vi "Test Report Contains Error Count.vi"(8 "error in (no error)":errorcluster, 11 "Text Report Test in":refnum<class "Text Report Test.lvclass">) -> (0 "error out":errorcluster, 3 "Text Report Test out":refnum<class "Text Report Test.lvclass">)   [LabVIEW 2020, in "Text Report Test.lvclass"]
uses:
  Text Report Test.lvclass
  Test Doubles/Test Case Test Double/Methods.ctl
  Text Report Test.lvclass/Text Report Test.ctl
  source/Plugins/Text Report/Text Report.lvclass
  Test Doubles/Test Case Test Double/Test Case Test Double.lvclass
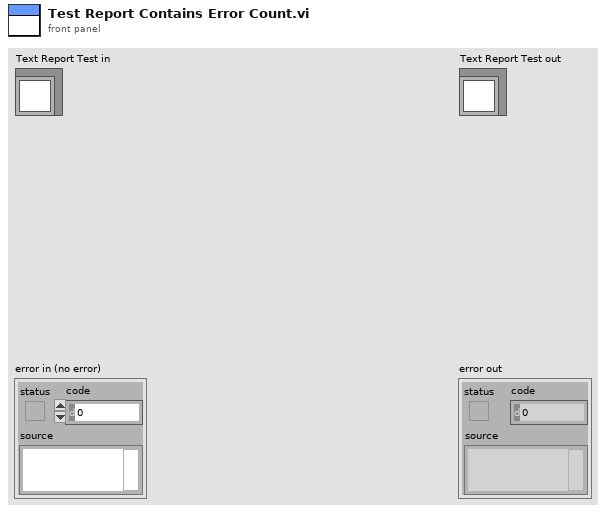
[diagram p1: front panel]
types:
  T1 = typedef "Test Case Test Double.lvclass/Methods.ctl" = enum16{"Test Failing Test.vi", "Test Passing Test.vi", "Test Error Test.vi", "Test Skip Test.vi", "Test Passing Pass If Test.vi", "Test Failing Pass If Test.vi", "Test Failing Fail If Test.vi", "Test Passing Fail If Test.vi", "Test Passing Pass If Error Test.vi", "Test Failing Pass If Error Test.vi", "Test Passing Fail If Error Test.vi", "Test Failing Fail If Error Test.vi", "Test Passing Pass If Equal Test.vi", "Test Failing Pass If Equal Test.vi", "Test Failing Fail If Equal Test.vi", "Test Passing Fail If Equal Test.vi", "Freezing Test.vi", "Test Pass on Expected Error Code.vi", "Test Error on Unexpected Error Code.vi", "Test Fail on Expected Error Code.vi", "Test Error when Fail on Unexpected Error Code.vi", "Test Pass on Expected Element in Array.vi", "Test Fail on Expected Element Not in Array.vi", "Test Pass on Expected Element in Set.vi", "Test Fail on Expected Element Not in Set.vi", "Test Pass on Expected Element in Map.vi", "Test Fail on Expected Element Not in Map.vi", "Test Fail on Unexpected Element in Array.vi", "Test Pass on Unexpected Element Not in Array.vi", "Test Fail if Unexpected Element in Set.vi", "Test Pass if Unexpected Element Not in Set.vi", "Test Fail if Unexpected Element in Map.vi", "Test Pass if Unexpected Element Not in Map.vi", "Test Pass on Expected Element in Array of Clusters.vi", "Test Pass on Expected Element Not in Array of Clusters.vi", "Test Matching String Test.vi", "Test Not Matching String Test.vi", "Verify Passing.vi", "Without Prefix.vi", "Private VI.vi"}
  T2 = typedef "Result.lvlib/Result.ctl" = cluster{"Name":string, "Description":string, "Status":T3, "Result Type":T4, "Execution Time":dbl, "Data":cluster{"Expected":variant, "Actual":variant, "Delta":variant}}
  T3 = typedef "Result.lvlib/Status.ctl" = enum16{"", "Passed", "Failed", "Error", "Skipped", "Setup Error", "Broken", "Teardown Error"}
  T4 = typedef "Result.lvlib/Type.ctl" = enum16{"Test Case", "Test Suite", "Test Run", "Pass", "Fail", "Skip", "Pass if", "Fail if", "Pass if Error", "Fail if Error", "Pass if Equal", "Fail if Equal"}
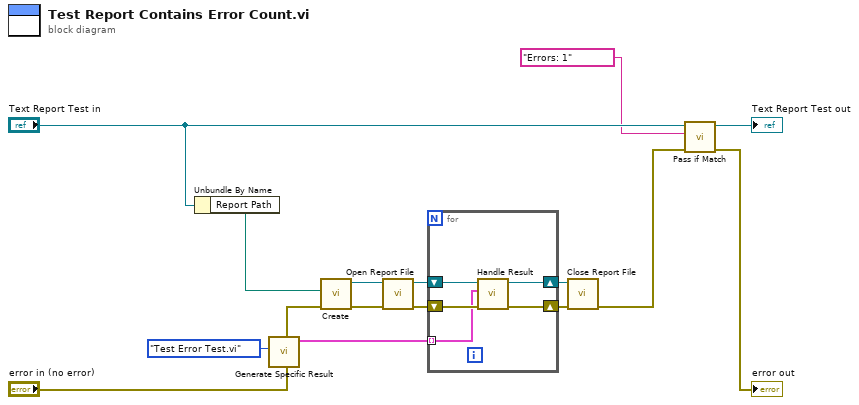
[diagram p0: block diagram]
diagram:
  n1 = Unbundle By Name("Text Report Test in") -> ("Report Path"=w1:path)
  n2 = call "Generate Specific Result.vi"("Test Method"=Methods."Test Error Test.vi") -> ("Data"=w6:T2[])  [unwired: 9 in, 1 out]
  n3 = call "Create.vi"("error in (no error)"="error in (no error)", "Report Path"=w1) -> ("error out"=w3:errorcluster, "Text Report"=w2:refnum<class "Text Report.lvclass">)  [unwired: 8 in]
  n4 = call-dynamic "Open Report File.vi"("error in (no error)"=w3, "Text Report In"=w2) -> ("error out"=w15:errorcluster, "Text Report Out"=w13:refnum<class "Text Report.lvclass">)  [unwired: 8 in]
  n5 = for {
    shift-right: [w19] -> w14
    shift-left: w15 -> [w20]
    shift-right: [w17] -> w12
    shift-left: w13 -> [w18]
    tunnel: w6 -> [w16] mode=indexing
    n6 = call-dynamic "Handle Result.vi"("error in (no error)"=w20, "Result"=w16, "Text Report In"=w18) -> ("error out"=w19:errorcluster, "Text Report Out"=w17:refnum<class "Text Report.lvclass">)  [unwired: 7 in]
  }
  n7 = call-dynamic "Close Report File.vi"("error in (no error)"=w14, "Text Report In"=w12) -> ("error out"=w7:errorcluster)  [unwired: 8 in, 1 out]
  n8 = call "Pass if Match.vi"("error in (no error)"=w7, "regular expression"="Errors: 1", "XML Report Test in"="Text Report Test in") -> ("error out"=→"error out":errorcluster, "XML Report Test out"=→"Text Report Test out":refnum<class "Text Report Test.lvclass">)  [unwired: 6 in, 1 out]
